vi "Call gRPC Wait.vi"(8 "error in (no error)":errorcluster, 10 "msec_to_wait":u64, 11 "address":string="localhost:50051") -> (0 "error out":errorcluster, 2 "timestamp":u64)   [LabVIEW 2021, in "gRPC Client Calls.lvlib"]
uses:
  gRPC Client Calls.lvlib
  test_service_client/RPC Messages/test_service_WaitRequest.ctl
  test_service_client/test_service_client.lvlib
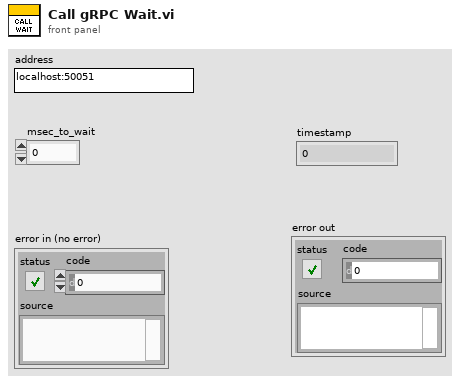
[diagram p1: front panel]
types:
  T1 = typedef "test_service_client.lvlib/test_service_WaitRequest.ctl" = cluster{"msec_to_wait":u64}
  T2 = typedef "grpc-lvsupport-release.lvlib/grpcId.ctl" = u64
  T3 = typedef "test_service_client.lvlib/test_service_WaitResponse.ctl" = cluster{"timestamp":u64}
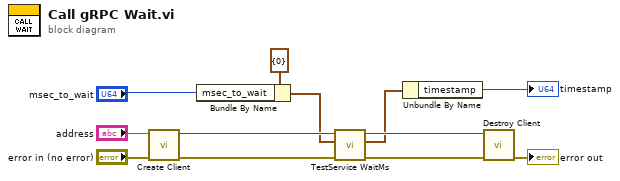
[diagram p0: block diagram]
diagram:
  n1 = call "Create Client.vi"("error in"="error in (no error)", "address"="address") -> ("error out"=w11:errorcluster, "gRPC ID Out"=w12:T2)  [unwired: 8 in]
  n2 = Bundle By Name(cluster=T1 {"msec_to_wait"=0} ("Request Data"), "msec_to_wait"="msec_to_wait") -> (w3:T1)
  n3 = call "TestService WaitMs.vi"("error in"=w11, "Request Data"=w3, "gRPC ID"=w12) -> ("error out"=w9:errorcluster, "Response Data"=w2:T3, "gRPC ID out"=w10:T2)  [unwired: 6 in]
  n4 = Unbundle By Name(w2) -> ("timestamp"=→"timestamp":u64)
  n5 = call "Destroy Client.vi"("error in"=w9, "gRPC ID"=w10) -> ("error out"=→"error out":errorcluster)  [unwired: 9 in]
